vi "RunProgramOnBrick.vi"(8 "error in (no error)":errorcluster, 10 "Program Name":string, 11 "VIA in":refnum<class "BotSpeak.lvclass">) -> (0 "error out":errorcluster, 3 "VIA out":refnum<class "BotSpeak.lvclass">)   [LabVIEW 2014, in "BotSpeak.lvclass"]
uses:
  <vilib>/NXT/LegoClasses/BotSpeak/BotSpeak.lvclass
panel:
  out "standard error":string
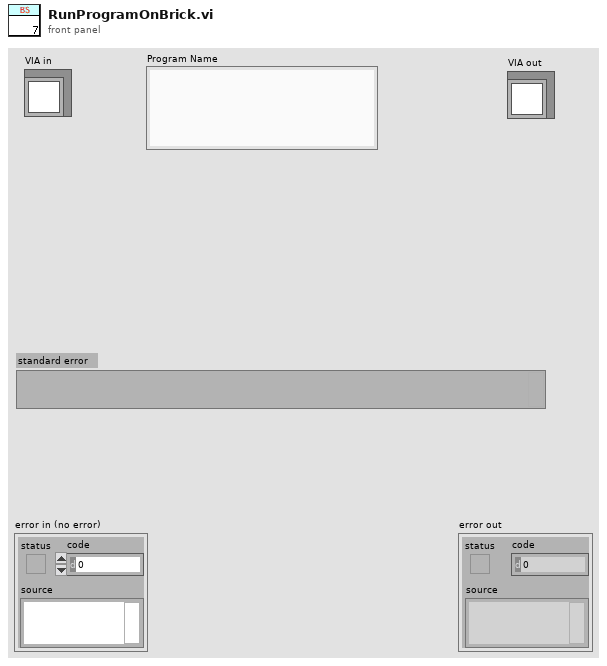
[diagram p1: front panel]
types:
  T1 = enum32{"Invalid", "Standard", "Closed", "Hidden", "Minimized", "Maximized"}
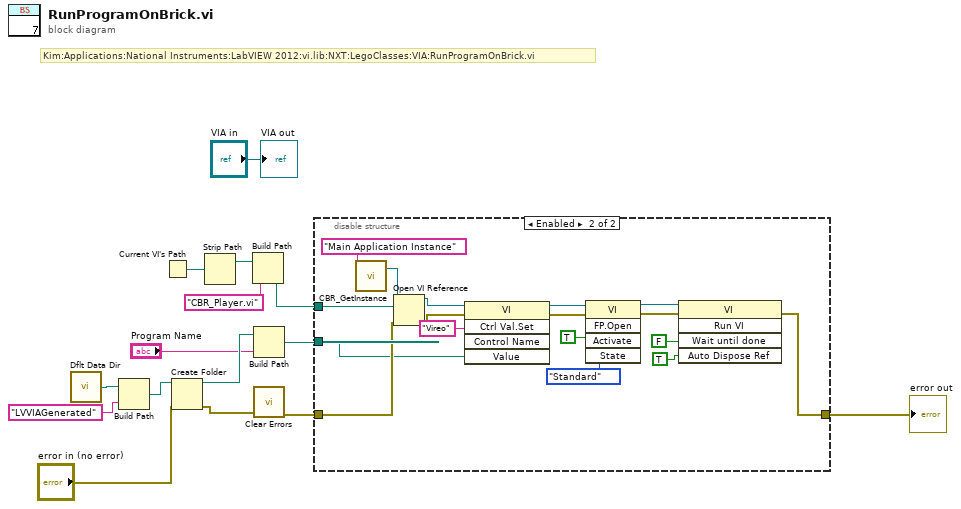
[diagram p0: block diagram]
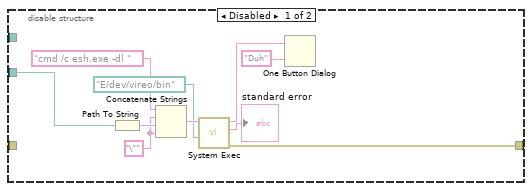
[diagram p2: hidden frame]
diagram:
  # "Kim:Applications:National Instruments:LabVIEW 2012:vi.lib:NXT:LegoClasses:VIA:RunProgramOnBrick.vi"
  n1 = call <vilib>:"Dflt Data Dir.vi"() -> ("App:Default Data Directory"=w15:path)
  n2 = Build Path(base path=w15, name or relative path="LVVIAGenerated" ("file (use dialog)")) -> (appended path=w14:path)
  n3 = Current VI's Path() -> (path=w6:path)
  n4 = Create Folder(path (use dialog)=w14, error in="error in (no error)") -> (created path=w9:path, error out=w12:errorcluster)  [unwired: 1 in, 1 out]
  n5 = Strip Path(path=w6) -> (stripped path=w5:path)  [unwired: 1 out]
  n6 = Build Path(base path=w5, name or relative path="CBR_Player.vi") -> (appended path=w4:path)
  n7 = Build Path(base path=w9, name or relative path="Program Name") -> (appended path=w8:path)
  n8 = call <vilib>:"Clear Errors.vi"("error in (no error)"=w12) -> ("error out"=w10:errorcluster)  [unwired: 5 in, 1 out]
  n9 = disable-structure shown="Enabled" {
    disable-tunnel: [w17 w29] -> w2
    disable-tunnel: w10 -> [_ w30]
    disable-tunnel: w8 -> [w16 w28]
    disable-tunnel: w4 -> [_ w27]
    frame Disabled {
      w24 = "\"" ("string")
      n10 = Path To String(path=w16) -> (string=w25:string)
      n11 = Concatenate Strings("cmd /c esh.exe -dl " ("string"), w24, w25, w24) -> (w21:string)
      n12 = call <vilib>:"System Exec.vi"("working directory"=path "E:/dev/vireo/bin" ("stripped path"), "command line"=w21) -> ("error out"=w17:errorcluster, "standard error"=→"standard error":string, "standard output"=w20:string)  [unwired: 6 in, 1 out]
      n13 = One Button Dialog(message=w20, button name ("OK")="Duh") -> ()  [unwired: 1 out]
    }
    frame Enabled {
      n14 = call <vilib>:"CBR_GetInstance.vi"("App.ContextName"="Main Application Instance") -> ("Application out"=w31:refnum<vi>)  [unwired: 2 in]
      n15 = Open VI Reference(application reference (local)=w31, vi path=w27, error in (no error)=w30) -> (vi reference=w36:refnum<vi>, error out=w35:errorcluster)  [unwired: 3 in]
      n16 = invoke class="VI" method="Ctrl Val.Set"(reference=w36, error in=w35, "Control Name"="Vireo", "Value"=w28) -> (reference out=w32:refnum<vi>, error out=w33:errorcluster)  [unwired: 1 in, 3 out]
      n17 = invoke class="VI" method="FP.Open"(reference=w32, error in=w33, "Activate"=TRUE ("Activate?"), "State"=T1."Standard") -> (reference out=w39:refnum<vi>, error out=w40:errorcluster)  [unwired: 1 in, 3 out]
      n18 = invoke class="VI" method="Run VI"(reference=w39, error in=w40, "Wait until done"=FALSE ("Wait Until Done"), "Auto Dispose Ref"=TRUE ("Wait Until Done")) -> (error out=w29:errorcluster)  [unwired: 1 in, 4 out]
    }
  }
  "error out" <- w2
  "VIA out" <- "VIA in"
